vi "Add Goal.vi"(5 "Month":T1, 7 "YYYY":i32, 8 "error in (no error)":errorcluster, 9 "Goal Amount":dbl, 10 "Category_id":i32, 11 "Database in":refnum<class "Database.lvclass">) -> (0 "error out":errorcluster, 3 "Database out":refnum<class "Database.lvclass">)   [LabVIEW 2018, in "Database.lvclass"]
uses:
  Database.lvclass
  Month.ctl
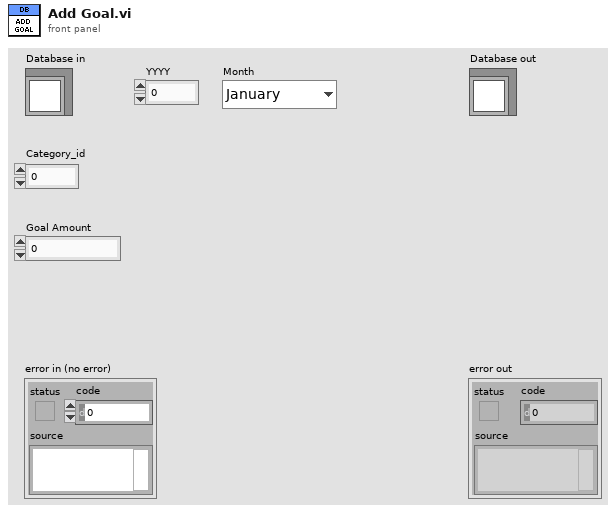
[diagram p1: front panel]
types:
  T1 = typedef "Database.lvclass/Month.ctl" = enum16{"January", "February", "March", "April", "May", "June", "July", "August", "September", "October", "November", "December"}
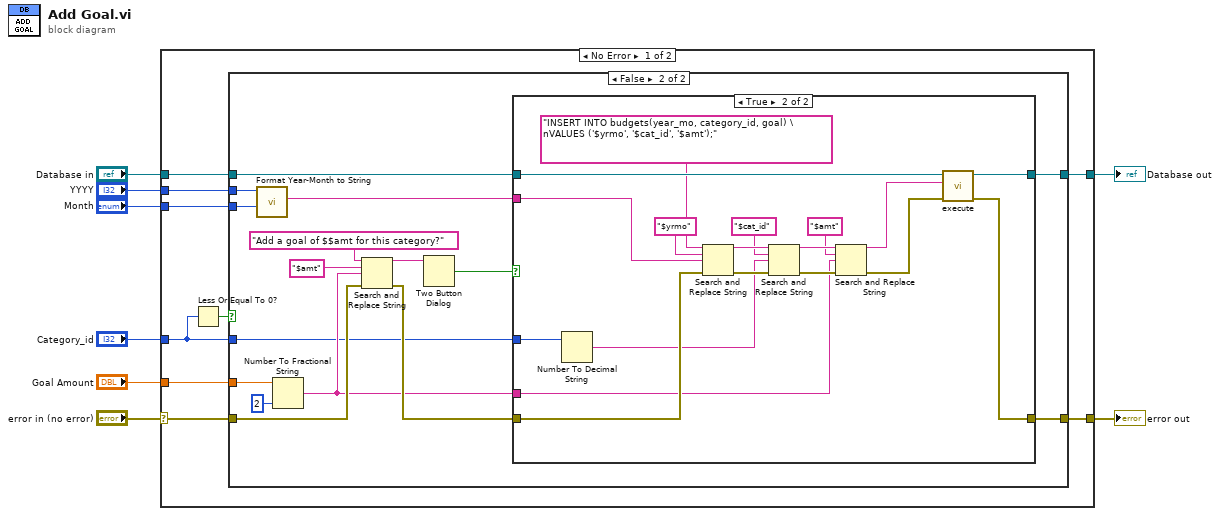
[diagram p0: block diagram]
diagram:
  n1 = case shown="No Error" "error in (no error)" {
    selector: "error in (no error)" -> [w13 w57]
    tunnel: [w15 w57] -> w7
    tunnel: [w16 w56] -> w5
    tunnel: "Database in" -> [w17 w56]
    tunnel: "Category_id" -> [w12 _]
    tunnel: "Goal Amount" -> [w14 _]
    tunnel: "YYYY" -> [w10 _]
    tunnel: "Month" -> [w9 _]
    frame No Error {
      n2 = Less Or Equal To 0?(x=w12) -> (x <= 0?=w11:bool)
      n3 = case shown="False" w11 {
        tunnel: w17 -> [w19 w35]
        tunnel: [w19 w34] -> w16
        tunnel: [w18 w33] -> w15
        tunnel: w14 -> [_ w32]
        tunnel: w13 -> [w18 w30]
        tunnel: w12 -> [_ w23]
        tunnel: w10 -> [_ w22]
        tunnel: w9 -> [_ w21]
        frame True {
        }
        frame False {
          n4 = call "Format Year-Month to String.vi"("Month"=w21, "YYYY"=w22) -> ("Year-Mo"=w20:string)  [unwired: 9 in]
          n5 = Number To Fractional String(number=w32, precision (6)=i16 2) -> (F-format string=w24:string)  [unwired: 2 in]
          n6 = Search and Replace String(input string="Add a goal of $$amt for this category?", search string="$amt", replace string=w24, error in=w30) -> (result string=w28:string, error out=w29:errorcluster)  [unwired: 4 in, 2 out]
          n7 = Two Button Dialog(message=w28) -> (T button?=w27:bool)  [unwired: 2 in]
          n8 = case shown="True" w27 {
            tunnel: w35 -> [w37 w55]
            tunnel: [w37 w54] -> w34
            tunnel: [w36 w53] -> w33
            tunnel: w29 -> [w36 w50]
            tunnel: w23 -> [_ w42]
            tunnel: w24 -> [_ w39]
            tunnel: w20 -> [_ w38]
            frame False {
            }
            frame True {
              n9 = Number To Decimal String(number=w42) -> (decimal integer string=w41:string)  [unwired: 1 in]
              n10 = Search and Replace String(input string="INSERT INTO budgets(year_mo, category_id, goal) \nVALUES ('$yrmo', '$cat_id', '$amt');", search string="$yrmo", replace string=w38, error in=w50) -> (result string=w49:string, error out=w48:errorcluster)  [unwired: 4 in, 2 out]
              n11 = Search and Replace String(input string=w49, search string="$cat_id", replace string=w41, error in=w48) -> (result string=w47:string, error out=w46:errorcluster)  [unwired: 4 in, 2 out]
              n12 = Search and Replace String(input string=w47, search string="$amt", replace string=w39, error in=w46) -> (result string=w40:string, error out=w45:errorcluster)  [unwired: 4 in, 2 out]
              n13 = call "execute.vi"("error in (no error)"=w45, "SQL query"=w40, "Database in"=w55) -> ("error out"=w53:errorcluster, "Database out"=w54:refnum<class "Database.lvclass">)  [unwired: 7 in]
            }
          }
        }
      }
    }
    frame Error {
    }
  }
  "error out" <- w7
  "Database out" <- w5
